vi "Set Data on Point.vi"(0 "eye scan point iterator":refnum<class "niHighSpeedSerial N Point Eye Scan Point Iterator v1 Host.lvclass">, 5 "bit error ratio":dbl, 7 "sample count":u64, 9 "error count":u64, 11 "error in":errorcluster) -> (4 "eye scan point iterator out":refnum<class "niHighSpeedSerial N Point Eye Scan Point Iterator v1 Host.lvclass">, 15 "error out":errorcluster)   [LabVIEW 2014, in "niHighSpeedSerial N Point Eye Scan Point Iterator v1 Host.lvclass"]
doc: "Sets the specified data on the active point.\n\n<B>Input Parameters</B>\n\n<B>eye scan point iterator</B> is the incoming wire for the Eye Scan Point Iterator class object\n\n<B>bit error rate</B> is the calculated statistical bit error rate based on the number of error counts and sample counts received.\n\n<B>sample count</B> is the number of samples that have been measured on this point.\n\n<B>error count</B> is the number of errors that have been measured on this point.\n\n<B>error in</B> describes error conditions that occur before this node runs. This input provides standard 'error in' functionality.\n\n<B>Output Parameters</B>\n\n<B>eye scan point iterator out</B> is the outgoing wire for the Eye Scan Point Iterator class object\n\n<B>error out</B> contains error information. This output provides standard 'error out' functionality."
uses:
  <instrlib>/niHighSpeedSerial/Eye Scan/v1/Host/Impl/N Pt Iter/niHighSpeedSerial N Point Eye Scan Point Iterator v1 Host.lvclass
  <instrlib>/niHighSpeedSerial/Eye Scan/v1/Host/Impl/N Pt Iter/niHighSpeedSerial N Point Eye Scan Point Iterator v1 Host.lvclass/niHighSpeedSerial N Point Eye Scan Point Iterator v1 Host.ctl
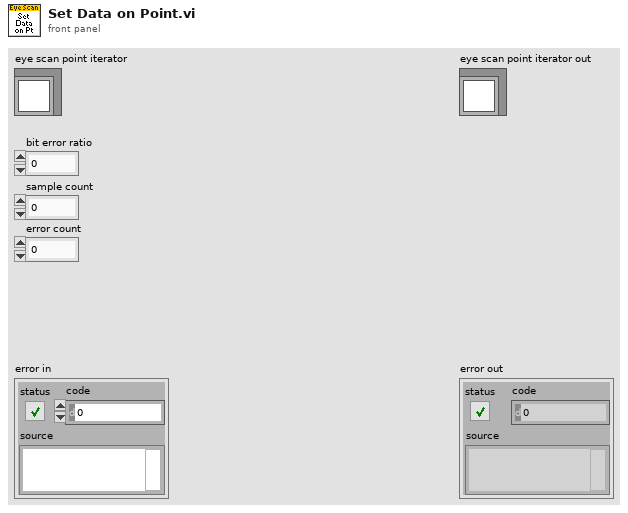
[diagram p1: front panel]
types:
  T1 = typedef "niHighSpeedSerial Eye Scan Common v1 Host.lvlib/Point.ctl" = cluster{"point offsets":T2, "sample count":u64, "error count":u64, "bit error ratio":dbl}
  T2 = typedef "niHighSpeedSerial Eye Scan Common v1 Host.lvlib/Point Offsets.ctl" = cluster{"horizontal offset":i16, "vertical offset":i8}
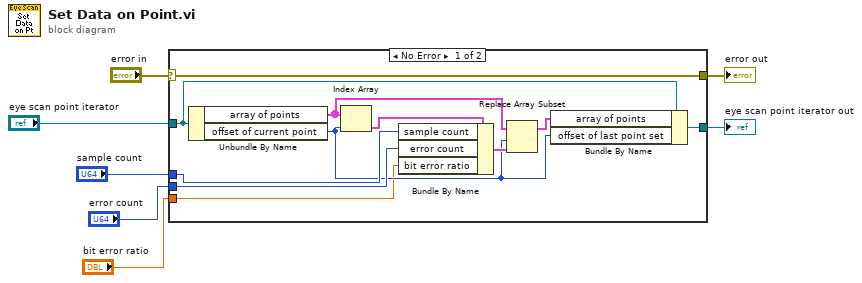
[diagram p0: block diagram]
diagram:
  n1 = case shown="No Error" "error in" {
    selector: "error in" -> [w16 w19]
    tunnel: [w10 w20] -> w7
    tunnel: "eye scan point iterator" -> [w11 w20]
    tunnel: [w16 w19] -> w4
    tunnel: "error count" -> [w17 _]
    tunnel: "sample count" -> [w18 _]
    tunnel: "bit error ratio" -> [w8 _]
    frame No Error {
      n2 = Unbundle By Name(w11) -> ("array of points"=w14:T1[], "offset of current point"=w9:i32)
      n3 = Index Array(array=w14, index=w9) -> (element=w15:T1)
      n4 = Bundle By Name(cluster=w15, "sample count"=w18, "error count"=w17, "bit error ratio"=w8) -> (w13:T1)
      n5 = Replace Array Subset(array=w14, new element=w13, index=w9) -> (w12:T1[])
      n6 = Bundle By Name(cluster=w11, "array of points"=w12, "offset of last point set"=w9) -> (w10:refnum<class "niHighSpeedSerial N Point Eye Scan Point Iterator v1 Host.lvclass">)
    }
    frame Error {
    }
  }
  "error out" <- w4
  "eye scan point iterator out" <- w7
